vi "MainRT.vi"() -> ()   [LabVIEW 2016]
panel:
  in  "error in (no error)":errorcluster
  out "error out":errorcluster
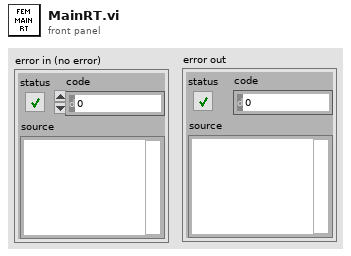
[diagram p1: front panel]
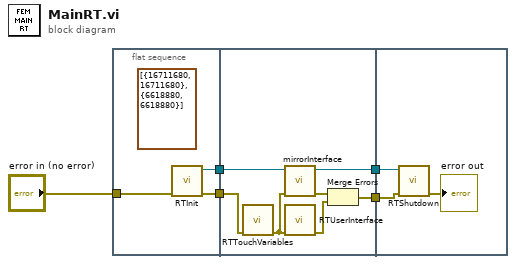
[diagram p0: block diagram]
diagram:
  n1 = flat-sequence {
    tunnel: [w8] -> w5
    tunnel: "error in (no error)" -> [w7]
    tunnel: [w6] -> w3
    tunnel: w5 -> [w10]
    tunnel: w3 -> [w15]
    tunnel: [w14] -> w2
    tunnel: [w13] -> w1
    tunnel: w2 -> [w17]
    tunnel: w1 -> [w16]
    frame #0 {
      (unwired) cluster{u32, u32}[] [{16711680, 16711680}, {6618880, 6618880}] ("Colors [4]")
      n2 = call "RTInit.vi"("error in (no error)"=w7) -> ("error out"=w8:errorcluster, "FPGA VI Reference Out"=w6:refnum<k20>)  [unwired: 9 in]
    }
    frame #1 {
      n3 = call "RTTouchVariables.vi"("error in (no error)"=w10) -> ("error out"=w9:errorcluster)  [unwired: 10 in]
      n4 = call "mirrorInterface.vi"("error in (no error)"=w9, "FPGA VI In"=w15) -> ("error out"=w11:errorcluster, "FPGA VI Reference Out"=w13:refnum<k20>)  [unwired: 8 in]
      n5 = call "RTUserInterface.vi"("error in (no error)"=w9) -> ("error out"=w12:errorcluster)  [unwired: 10 in]
      n6 = Merge Errors(w11, w12) -> (w14:errorcluster)
    }
    frame #2 {
      n7 = call "RTShutdown.vi"("FPGA VI Reference In"=w16, "error in (no error)"=w17) -> ("error out"=→"error out":errorcluster)  [unwired: 8 in]
    }
  }
